vi "Five_Blinking_Lights.vi"() -> ()   [LabVIEW 2022 SP3]
panel:
  in  "?":bool
  out "1":bool
  out "2":bool
  out "3":bool
  out "4":bool
  out "0":bool
  # "Five_Blinking_Lights:\nThe 5 lights will blink for one second each, until stopped.\nAt this point, the lights will continue until the final light has\nbeen extinguished."
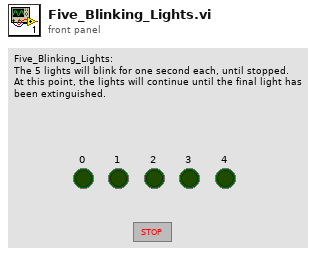
[diagram p1: front panel]
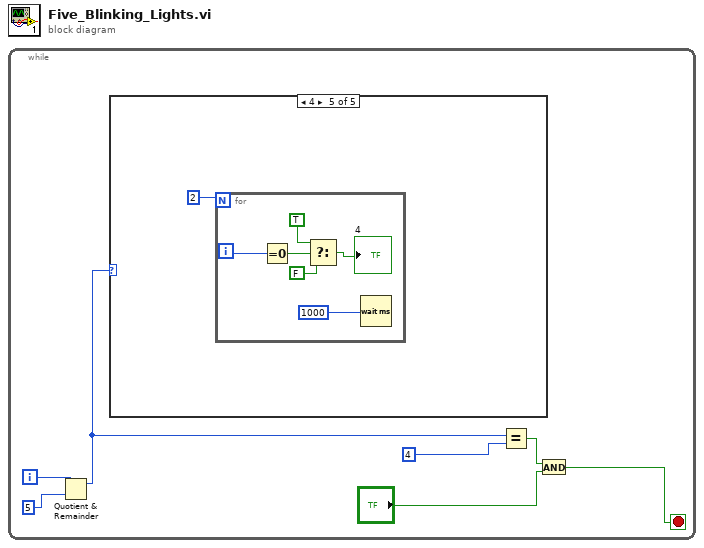
[diagram p0: block diagram]
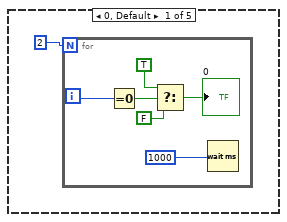
[diagram p2: hidden frame]
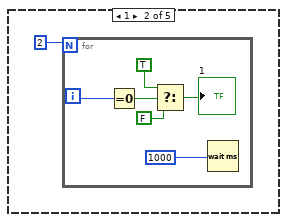
[diagram p3: hidden frame]
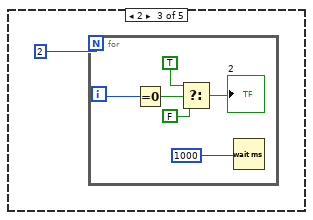
[diagram p4: hidden frame]
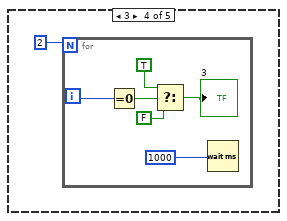
[diagram p5: hidden frame]
diagram:
  n1 = while {
    i -> [w7]
    stop <- w1 stop-if-true
    n2 = Quotient & Remainder(x=w7, y=5) -> (x-y*floor(x/y)=w5:i32)  [unwired: 1 out]
    n3 = case shown="4" w5 {
      frame 0, Default {
        n4 = for {
          N: 2 -> [_]
          i -> [w10]
          n5 = Equal To 0?(x=w10) -> (x = 0?=w11:bool)
          n6 = Select(t=TRUE, s=w11, f=FALSE) -> (s? t:f=→"0":bool)
          n7 = Wait (ms)(milliseconds to wait=1000) -> ()  [unwired: 1 out]
        }
      }
      frame 1 {
        n8 = for {
          N: 2 -> [_]
          i -> [w17]
          n9 = Equal To 0?(x=w17) -> (x = 0?=w18:bool)
          n10 = Select(t=TRUE, s=w18, f=FALSE) -> (s? t:f=→"1":bool)
          n11 = Wait (ms)(milliseconds to wait=1000) -> ()  [unwired: 1 out]
        }
      }
      frame 2 {
        n12 = for {
          N: 2 -> [_]
          i -> [w24]
          n13 = Equal To 0?(x=w24) -> (x = 0?=w25:bool)
          n14 = Select(t=TRUE, s=w25, f=FALSE) -> (s? t:f=→"2":bool)
          n15 = Wait (ms)(milliseconds to wait=1000) -> ()  [unwired: 1 out]
        }
      }
      frame 3 {
        n16 = for {
          N: 2 -> [_]
          i -> [w31]
          n17 = Equal To 0?(x=w31) -> (x = 0?=w32:bool)
          n18 = Select(t=TRUE, s=w32, f=FALSE) -> (s? t:f=→"3":bool)
          n19 = Wait (ms)(milliseconds to wait=1000) -> ()  [unwired: 1 out]
        }
      }
      frame 4 {
        n20 = for {
          N: 2 -> [_]
          i -> [w38]
          n21 = Equal To 0?(x=w38) -> (x = 0?=w39:bool)
          n22 = Select(t=TRUE, s=w39, f=FALSE) -> (s? t:f=→"4":bool)
          n23 = Wait (ms)(milliseconds to wait=1000) -> ()  [unwired: 1 out]
        }
      }
    }
    n24 = Equal?(x=w5, y=4) -> (x = y?=w3:bool)
    n25 = And(x=w3, y="?") -> (x .and. y?=w1:bool)
  }
